vi "Rename.vi"(8 "error in (no error)":errorcluster, 9 "New name":string, 10 "ProjectItem Refnum":refnum<vi>, 11 "EXE in":refnum<class "NI_AB_API_EXE.lvclass">) -> (0 "error out":errorcluster, 3 "EXE out":refnum<class "NI_AB_API_EXE.lvclass">)   [LabVIEW 2020, in "NI_AB_API_EXE.lvclass"]
uses:
  <vilib>/AppBuilder/AB_API/EXE/NI_AB_API_EXE.lvclass
  <vilib>/AppBuilder/AB_API/Application/NI_AB_API_Application.lvclass
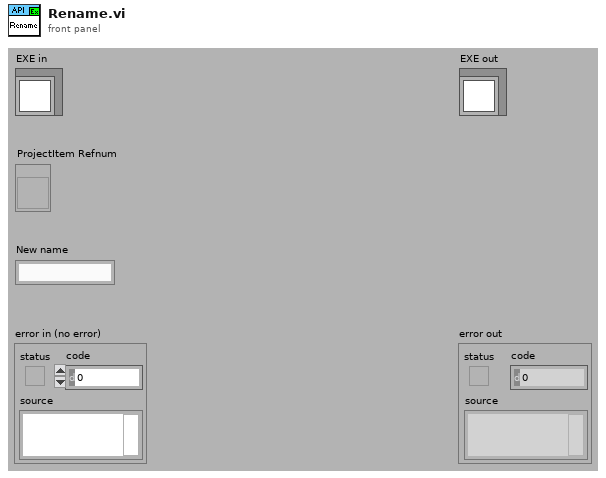
[diagram p1: front panel]
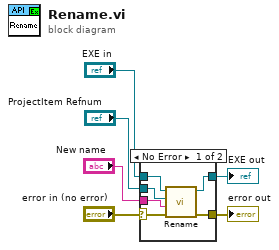
[diagram p0: block diagram]
diagram:
  n1 = case shown="No Error" "error in (no error)" {
    selector: "error in (no error)" -> [w9 w14]
    tunnel: [w10 w14] -> w5
    tunnel: [w11 w13] -> w3
    tunnel: "EXE in" -> [w12 w13]
    tunnel: "New name" -> [w8 _]
    tunnel: "ProjectItem Refnum" -> [w7 _]
    frame No Error {
      n2 = call-parent "Rename.vi"("error in (no error)"=w9, "New name"=w8, "ProjectItem Refnum"=w7, "Build in"=w12) -> ("error out"=w10:errorcluster, "Build out"=w11:refnum<class "NI_AB_API_EXE.lvclass">)  [unwired: 6 in]
    }
    frame Error {
    }
  }
  "error out" <- w5
  "EXE out" <- w3
